vi "WriteAlarms.vi"(8 "ErrorIn":errorcluster, 10 "Alarms":refnum<class "IAlarm.lvclass">[](array[class]), 11 "IActionIn":refnum<class "IAction.lvclass">) -> (0 "ErrorOut":errorcluster, 3 "IActionOut":refnum<class "IAction.lvclass">)   [LabVIEW 2019]
uses:
  IAction.lvclass
  Alarm/IAlarm.lvclass
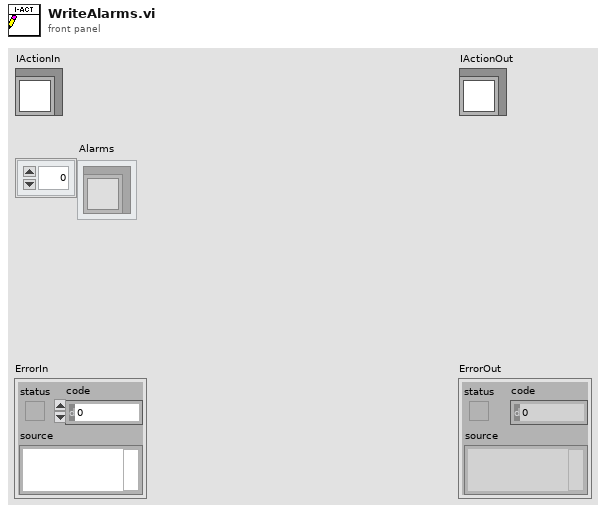
[diagram p1: front panel]
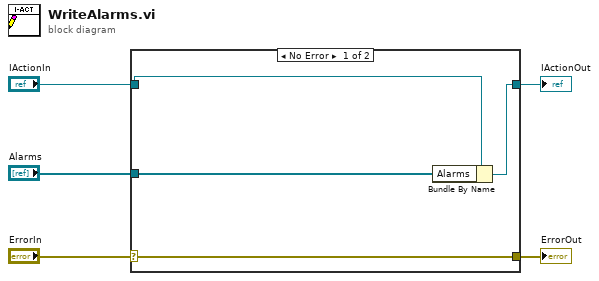
[diagram p0: block diagram]
diagram:
  n1 = case shown="No Error" "ErrorIn" {
    selector: "ErrorIn" -> [w9 w10]
    tunnel: [w9 w10] -> w4
    tunnel: [w7 w11] -> w2
    tunnel: "IActionIn" -> [w8 w11]
    tunnel: "Alarms" -> [w6 _]
    frame No Error {
      n2 = Bundle By Name(cluster=w8, "Alarms"=w6) -> (w7:refnum<class "IAction.lvclass">)
    }
    frame Error {
    }
  }
  "ErrorOut" <- w4
  "IActionOut" <- w2
